vi "SDSU_MemRange.vi"(10 "memin":string) -> (1 "inc adds":bool, 2 "address":i32[](array[numeric]) format="%x", 3 "remaining string":string)   [LabVIEW 2016]
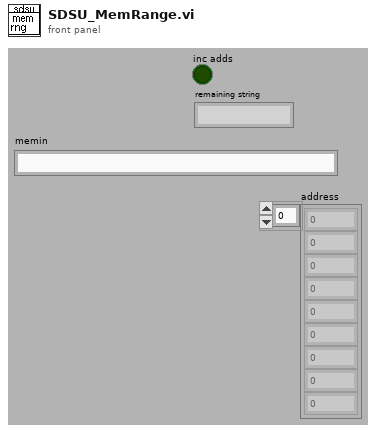
[diagram p1: front panel]
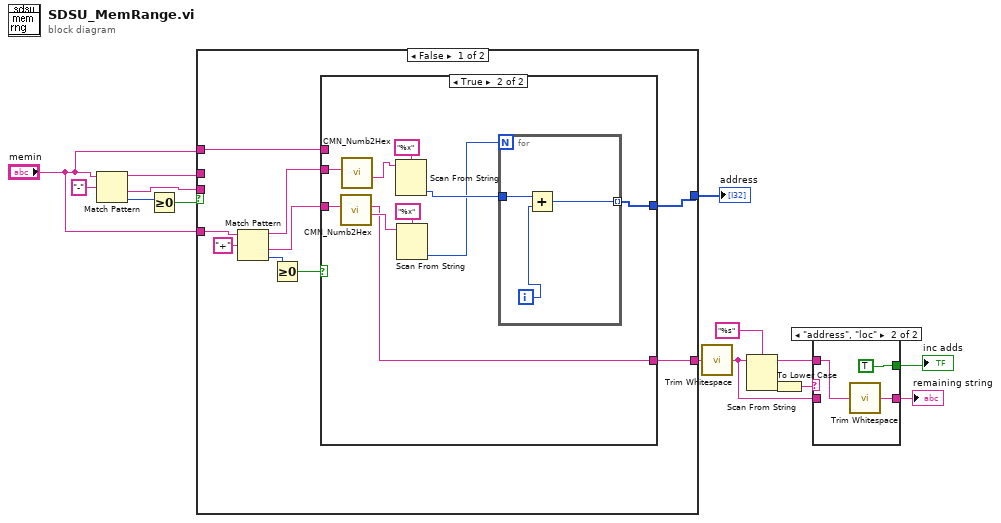
[diagram p0: block diagram]
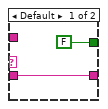
[diagram p2: hidden frame]
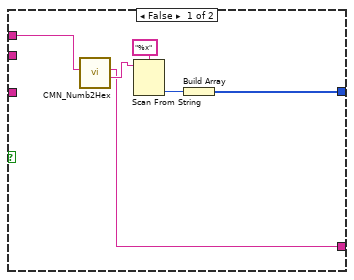
[diagram p3: hidden frame]
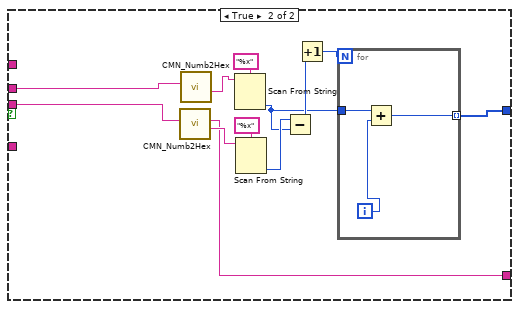
[diagram p4: hidden frame]
diagram:
  n1 = Match Pattern(string="memin", regular expression="-") -> (before substring=w11:string, after substring=w12:string, offset past match=w14:i32)  [unwired: 2 out]
  n2 = Greater Or Equal To 0?(x=w14) -> (x >= 0?=w13:bool)
  n3 = case shown="False" w13 {
    tunnel: "memin" -> [w24 _]
    tunnel: w12 -> [_ w55]
    tunnel: w11 -> [_ w54]
    tunnel: [w23 w46] -> w10
    tunnel: [w22 w44] -> w8
    tunnel: "memin" -> [w17 _]
    frame False {
      n4 = Match Pattern(string=w17, regular expression="+") -> (before substring=w19:string, after substring=w18:string, offset past match=w21:i32)  [unwired: 2 out]
      n5 = Greater Or Equal To 0?(x=w21) -> (x >= 0?=w16:bool)
      n6 = case shown="True" w16 {
        tunnel: w24 -> [w28 _]
        tunnel: [w26 w32] -> w23
        tunnel: [w25 w31] -> w22
        tunnel: w19 -> [_ w35]
        tunnel: w18 -> [_ w34]
        frame False {
          n7 = call "CMN_Numb2Hex.vi"("input str"=w28) -> ("output hexa"=w29:string, "remaining string"=w25:string)  [unwired: 9 out]
          n8 = Scan From String(format string="%x" ("Format String"), input string=w29) -> (output 1=w27:u32)  [unwired: 2 in, 4 out]
          n9 = Build Array(w27) -> (w26:u32[])
        }
        frame True {
          n10 = call "CMN_Numb2Hex.vi"("input str"=w34) -> ("output hexa"=w37:string, "remaining string"=w31:string)  [unwired: 9 out]
          n11 = call "CMN_Numb2Hex.vi"("input str"=w35) -> ("output hexa"=w39:string)  [unwired: 10 out]
          n12 = Scan From String(format string="%x" ("Format String"), input string=w39) -> (output 1=w36:u32)  [unwired: 2 in, 4 out]
          n13 = Scan From String(format string="%x" ("Format String"), input string=w37) -> (output 1=w33:u32)  [unwired: 2 in, 4 out]
          n14 = for {
            N: w33 -> [_]
            tunnel: w36 -> [w43]
            tunnel: [w41] -> w32 mode=indexing
            i -> [w42]
            n15 = Add(x=w43, y=w42) -> (x+y=w41:u32)
          }
        }
      }
    }
    frame True {
      n16 = call "CMN_Numb2Hex.vi"("input str"=w55) -> ("output hexa"=w50:string, "remaining string"=w44:string)  [unwired: 9 out]
      n17 = call "CMN_Numb2Hex.vi"("input str"=w54) -> ("output hexa"=w52:string)  [unwired: 10 out]
      n18 = Scan From String(format string="%x" ("Format String"), input string=w52) -> (output 1=w47:u32)  [unwired: 2 in, 4 out]
      n19 = Scan From String(format string="%x" ("Format String"), input string=w50) -> (output 1=w49:u32)  [unwired: 2 in, 4 out]
      n20 = Subtract(x=w49, y=w47) -> (x-y=w48:u32)
      n21 = Increment(x=w48) -> (x+1=w45:u32)
      n22 = for {
        N: w45 -> [_]
        tunnel: w47 -> [w58]
        tunnel: [w56] -> w46 mode=indexing
        i -> [w57]
        n23 = Add(x=w58, y=w57) -> (x+y=w56:u32)
      }
    }
  }
  "address" <- w10
  n24 = call <vilib>:"Trim Whitespace.vi"("string"=w8) -> ("trimmed string"=w6:string)  [unwired: 1 in]
  n25 = Scan From String(format string="%s", input string=w6) -> (remaining string=w2:string, output 1=w5:string)  [unwired: 2 in, 3 out]
  n26 = To Lower Case(string=w5) -> (all lower case string=w3:string)
  n27 = case shown="\"address\", \"loc\"" w3 {
    tunnel: [FALSE TRUE] -> w9
    tunnel: w6 -> [w59 _]
    tunnel: [w59 w61] -> w7
    tunnel: w2 -> [_ w62]
    frame Default {
    }
    frame "address", "loc" {
      n28 = call <vilib>:"Trim Whitespace.vi"("string"=w62) -> ("trimmed string"=w61:string)  [unwired: 1 in]
    }
  }
  "inc adds" <- w9
  "remaining string" <- w7
